vi "Off.vi"(8 "error in (no error)":errorcluster, 11 "BiStableShutter in":refnum<class "BiStableShutter.lvclass">) -> (0 "error out":errorcluster, 3 "BiStableShutter out":refnum<class "BiStableShutter.lvclass">)   [LabVIEW 2016, in "BiStableShutter.lvclass"]
uses:
  BiStableShutter.lvclass
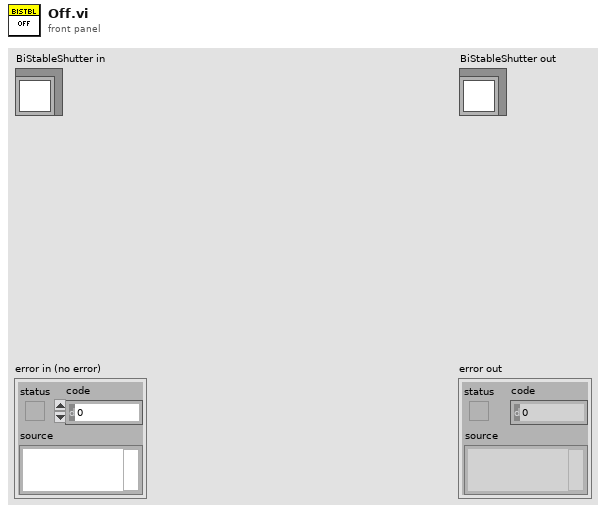
[diagram p1: front panel]
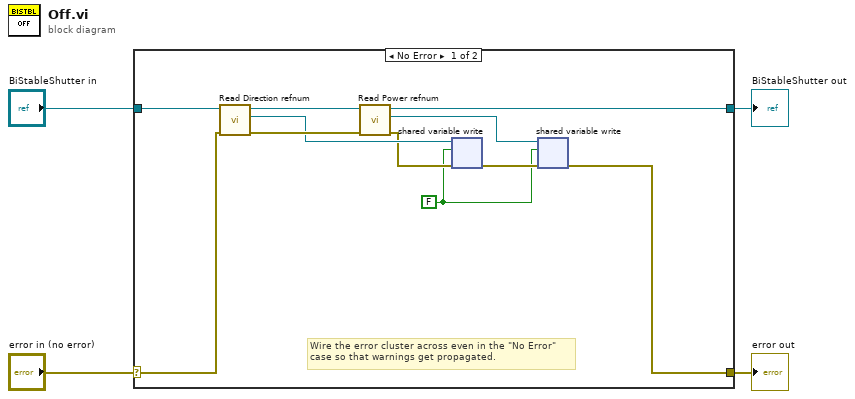
[diagram p0: block diagram]
diagram:
  n1 = case shown="No Error" "error in (no error)" {
    selector: "error in (no error)" -> [w6 w17]
    tunnel: [w5 w17] -> w3
    tunnel: [w8 w16] -> w1
    tunnel: "BiStableShutter in" -> [w7 w16]
    frame No Error {
      w9 = FALSE
      # "Wire the error cluster across even in the \"No Error\"\ncase so that warnings get propagated."
      n2 = call-dynamic "Read Direction refnum.vi"("error in (no error)"=w6, "BiStableShutter in"=w7) -> ("error out"=w14:errorcluster, "Direction refnum"=w13:refnum<k21>, "BiStableShutter out"=w15:refnum<class "BiStableShutter.lvclass">)  [unwired: 7 in]
      n3 = call-dynamic "Read Power refnum.vi"("error in (no error)"=w14, "BiStableShutter in"=w15) -> ("error out"=w11:errorcluster, "Power refnum"=w12:refnum<k21>, "BiStableShutter out"=w8:refnum<class "BiStableShutter.lvclass">)  [unwired: 7 in]
      n4 = shared-variable-write(w13, w11, w9) -> (w10:errorcluster)  [unwired: 1 out]
      n5 = shared-variable-write(w12, w10, w9) -> (w5:errorcluster)  [unwired: 1 out]
    }
    frame Error {
    }
  }
  "error out" <- w3
  "BiStableShutter out" <- w1
